vi "InstrumentControlMaster.vi"() -> ()   [LabVIEW 2019]
panel:
  out "error out":errorcluster
  out "call:outputs":T1(array[cluster]) {"type\ndescriptor" format="%.0x"}
  out "get state:window state":enum32{"Closed", "Open", "Open and Active"}(ring)
  out "get state:vi state":enum32{"Broken", "Idle", "Running"}(ring)
  in  "open:use VI Setup settings":bool=TRUE
  in  "set size:panel location and size":T2
  in  "error in (no error)":errorcluster
  in  "call:retrieve all outputs (F:only specified)\nclose:use old abort on close behavior(T)":bool
  in  "call:mode (open,call,close:1)":T3(ring)=enum."open panel, call VI, close panel if originally closed"
  in  "call:desired outputs":T1(array[cluster]) {"type\ndescriptor" format="%.0x"}
  in  "call:inputs":T1(array[cluster]) {"type\ndescriptor" format="%.0x"}
  in  "Load:VI path":path
  in  "all ops:VI name":string
  in  "operation":T4(ring)
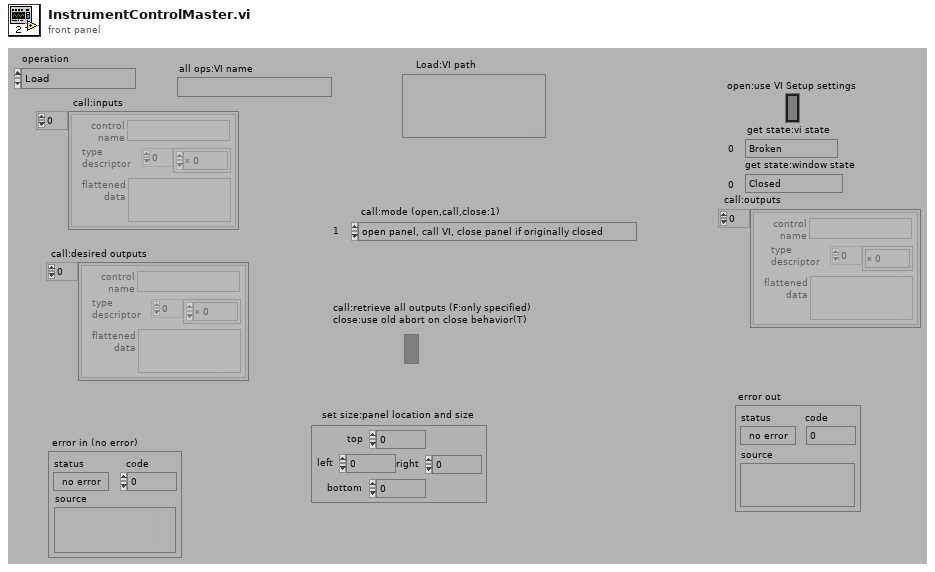
[diagram p1: front panel]
types:
  T1 = cluster{"control\nname":string, "type\ndescriptor":i16[], "flattened\ndata":string}[]
  T2 = cluster{"top":i16, "left":i16, "bottom":i16, "right":i16}
  T3 = enum16{"call as is", "open panel, call VI, close panel if originally closed"}
  T4 = enum16{"Load", "Call", "Release", "Size FP", "Open FP", "Close FP", "Run", "Get VI State", "Get FP Size", "Abort"}
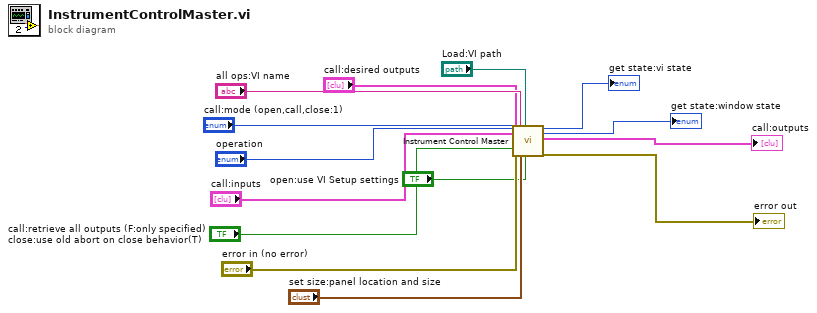
[diagram p0: block diagram]
diagram:
  n1 = call <vilib>:"Instrument Control Master.vi"("operation"="operation", "call:inputs"="call:inputs", "call:desired outputs"="call:desired outputs", "call:mode (open,call,close:1)"="call:mode (open,call,close:1)", "call:retrieve all outputs (F:only specified)\nclose:use old abort on close behavior(T)"="call:retrieve all outputs (F:only specified)\nclose:use old abort on close behavior(T)", "error in (no error)"="error in (no error)", "all ops:VI name"="all ops:VI name", "set size:panel location and size"="set size:panel location and size", "Load:VI path"="Load:VI path", "open:use VI Setup settings"="open:use VI Setup settings") -> ("get state:vi state"=→"get state:vi state":enum32{"Broken", "Idle", "Running"}, "get state:window state"=→"get state:window state":enum32{"Closed", "Open", "Open and Active"}, "call:outputs"=→"call:outputs":T1, "error out"=→"error out":errorcluster)  [unwired: 5 in, 1 out]
